vi "util_create_folder_recursive.vi"(8 "error in":errorcluster, 11 "path in":path) -> (0 "error out":errorcluster, 3 "path out":path)   [LabVIEW 2015, in "lv-bin.lvlib" / "v1.lvlib"]
uses:
  v1.lvlib
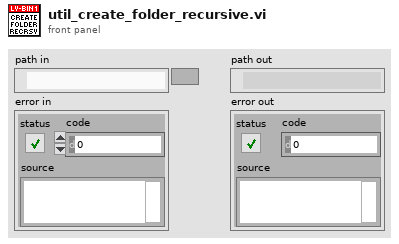
[diagram p1: front panel]
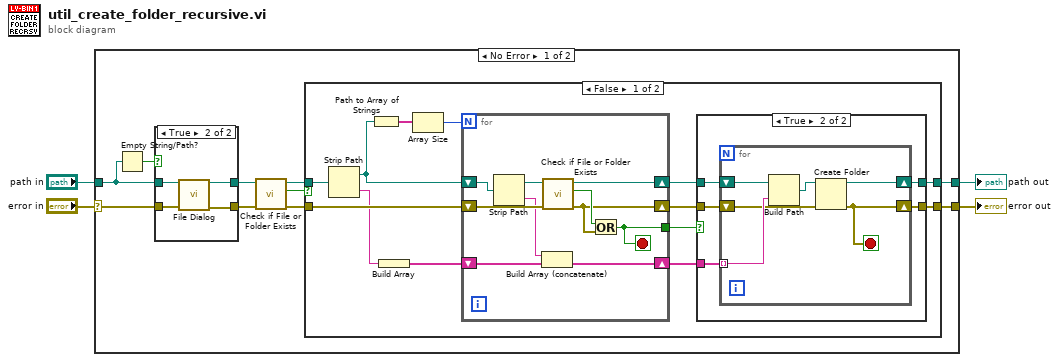
[diagram p0: block diagram]
diagram:
  n1 = case shown="No Error" "error in" {
    selector: "error in" -> [w12 w58]
    tunnel: "path in" -> [w14 _]
    tunnel: [w6 w58] -> w2
    tunnel: [w5 _] -> w1
    frame No Error {
      n2 = Empty String/Path?(string/path=w14) -> (empty?=w13:bool)
      n3 = case shown="True" w13 {
        tunnel: w14 -> [w53 w57]
        tunnel: [w53 w56] -> w11
        tunnel: w12 -> [w52 w55]
        tunnel: [w52 w54] -> w10
        frame False {
        }
        frame True {
          n4 = call "File Dialog"("start path"=w57, "error in"=w55) -> ("selected path"=w56:path, "error out"=w54:errorcluster)  [unwired: 10 in, 2 out]
        }
      }
      n5 = call <vilib>:"Check if File or Folder Exists.vi"("error in (no error)"=w10, "path"=w11) -> ("error out"=w8:errorcluster, "file or folder exists?"=w7:bool, "dup path"=w9:path)  [unwired: 7 in]
      n6 = case shown="False" w7 {
        tunnel: w9 -> [w24 w50]
        tunnel: w8 -> [w25 w51]
        tunnel: [w16 w51] -> w6
        tunnel: [w15 w50] -> w5
        frame False {
          n7 = Strip Path(path=w24) -> (stripped path=w21:path, name=w23:string)
          n8 = Path to Array of Strings(0:w21) -> (2:w27:string[])  [unwired: 1 out]
          n9 = Build Array(w23) -> (w22:string[])
          n10 = Array Size(array=w27) -> (size(s)=w26:i32)
          n11 = for {
            N: w26 -> [_]
            shift-right: [w49] -> w19
            shift-left: w21 -> [w45]
            shift-right: [w46] -> w18
            shift-left: w25 -> [w48]
            tunnel: [w43] -> w20
            shift-right: [w42] -> w17
            shift-left: w22 -> [w41]
            stop <- w43 stop-if-true
            n12 = Strip Path(path=w45) -> (stripped path=w44:path, name=w40:string)
            n13 = Build Array (concatenate)(w40, w41) -> (w42:string[])
            n14 = call <vilib>:"Check if File or Folder Exists.vi"("error in (no error)"=w48, "path"=w44) -> ("error out"=w46:errorcluster, "file or folder exists?"=w47:bool, "dup path"=w49:path)  [unwired: 7 in]
            n15 = Or(x=w47, y=w46) -> (x .or. y?=w43:bool)
          }
          n16 = case shown="True" w20 {
            tunnel: w19 -> [_ w32]
            tunnel: w18 -> [w28 w31]
            tunnel: w17 -> [_ w33]
            tunnel: [w28 w29] -> w16
            tunnel: [_ w30] -> w15
            frame False {
            }
            frame True {
              n17 = for {
                tunnel: w33 -> [w38] mode=indexing
                shift-right: [w34] -> w30
                shift-left: w32 -> [w39]
                shift-right: [w35] -> w29
                shift-left: w31 -> [w37]
                stop <- w35 stop-if-true
                n18 = Build Path(base path=w39, name or relative path=w38) -> (appended path=w36:path)
                n19 = Create Folder(path (use dialog)=w36, error in=w37) -> (created path=w34:path, error out=w35:errorcluster)  [unwired: 1 in, 1 out]
              }
            }
          }
        }
        frame True {
        }
      }
    }
    frame Error {
    }
  }
  "error out" <- w2
  "path out" <- w1
